vi "Perform Action DataSocket Reply.vi"(6 "DataSocket Reply URL":string, 8 "error in":errorcluster, 9 "Input":variant, 10 "Task-Point Ident":string, 11 "IMSS Target Actor in":refnum<class "IMSS Target Actor.lvclass">) -> (0 "error out":errorcluster, 3 "IMSS Target Actor out":refnum<class "IMSS Target Actor.lvclass">)   [LabVIEW 2024, in "IMSS Target Actor.lvlib" / "IMSS Target Actor.lvclass"]
uses:
  IMSS Target Actor.lvclass
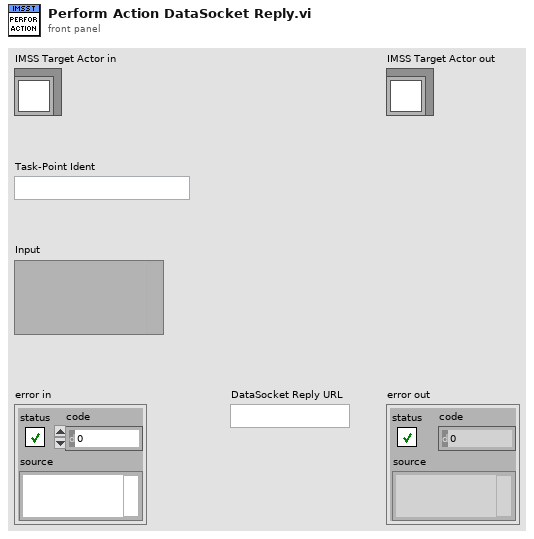
[diagram p1: front panel]
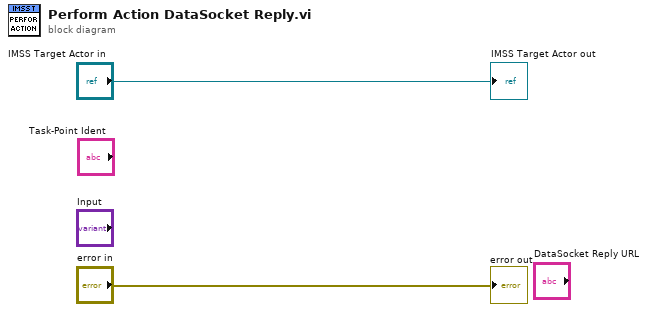
[diagram p0: block diagram]
diagram:
  "error out" <- "error in"
  "IMSS Target Actor out" <- "IMSS Target Actor in"
